vi "Get Object Parameter - Numeric.vi"(8 "error in (no error)":errorcluster, 9 "Default Value if JSON Null":dbl, 10 "Parameter Name":string, 11 "JSON Tree In (JSON Object)":variant) -> (0 "error out":errorcluster, 1 "is JSON Null?":bool, 2 "Double Value":dbl, 3 "JSON Tree Out Passthrough":variant)   [LabVIEW 2011, in "i3-json.lvlib"]
doc: "Use this template to build a VI to use as a subVI."
uses:
  i3-json.lvlib
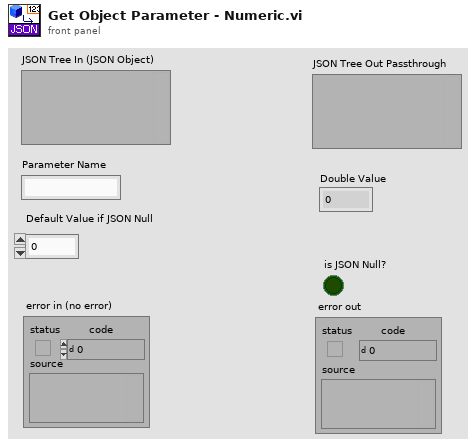
[diagram p1: front panel]
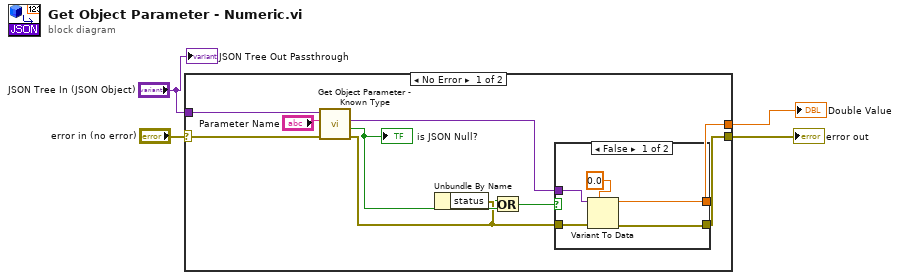
[diagram p0: block diagram]
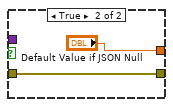
[diagram p2: hidden frame]
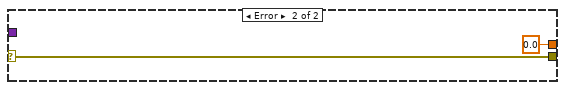
[diagram p3: hidden frame]
diagram:
  n1 = case shown="No Error" "error in (no error)" {
    selector: "error in (no error)" -> [w13 w23]
    tunnel: [w11 w23] -> w3
    tunnel: "JSON Tree In (JSON Object)" -> [w14 _]
    tunnel: [w8 0.0 ("Default Value if JSON Null")] -> w2
    frame No Error {
      n2 = call "Get Object Parameter - Known Type.vi"("error in (no error)"=w13, "Parameter Name"="Parameter Name", "JSON Tree In (JSON Object)"=w14) -> ("error out"=w6:errorcluster, "is JSON Null?"=w9:bool, "Value"=w10:variant)  [unwired: 3 in, 3 out]
      "is JSON Null?" <- w9
      n3 = Unbundle By Name(w6) -> ("status"=w5:bool)
      n4 = Or(x=w5, y=w9) -> (x .or. y?=w12:bool)
      n5 = case shown="False" w12 {
        tunnel: w6 -> [w19 w21]
        tunnel: [w16 w21] -> w11
        tunnel: w10 -> [w18 _]
        tunnel: [w17 "Default Value if JSON Null"] -> w8
        frame False {
          n6 = Variant To Data(error in=w19, type=0.0 ("Double Value"), Variant=w18) -> (data=w17:dbl, error out=w16:errorcluster)
        }
        frame True {
        }
      }
    }
    frame Error {
    }
  }
  "error out" <- w3
  "Double Value" <- w2
  "JSON Tree Out Passthrough" <- "JSON Tree In (JSON Object)"
